vi "catch_block_on_floor.vi"() -> ()   [LabVIEW 2013]
panel:
  out "Voltage":dbl(graph)
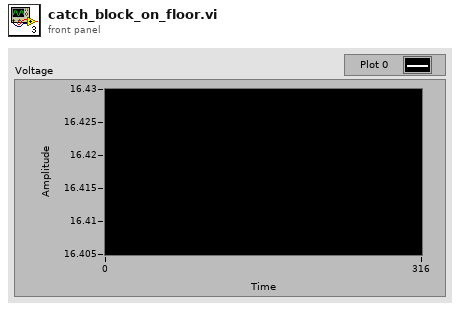
[diagram p1: front panel]
types:
  T1 = typedef "KNR3 Reference.ctl" = cluster{"FPGA Session":refnum<class "FPGA Interface Base.lvclass">, "Resource":T2}
  T2 = typedef "Resource.ctl" = enum16{"KNRm_DDRC", "KNRm_DDDD", "KNRm_DDDR", "KNRm_DDDC", "KNR"}
  T3 = cluster{"Mode":enum16{"FRWD", "TURFIX", "TURNOF"}, "Dir":enum16{"Left", "Right"}, "Pcmd":dbl, "Vcmd":dbl}
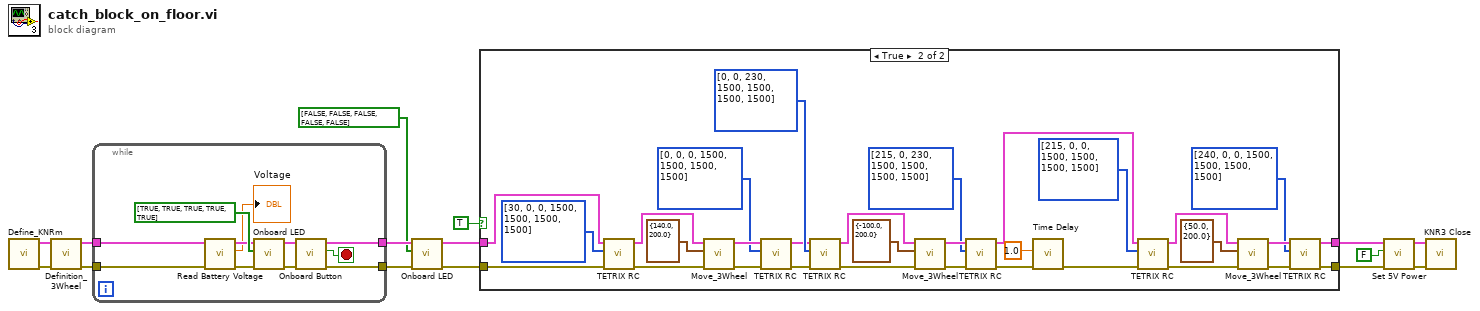
[diagram p0: block diagram]
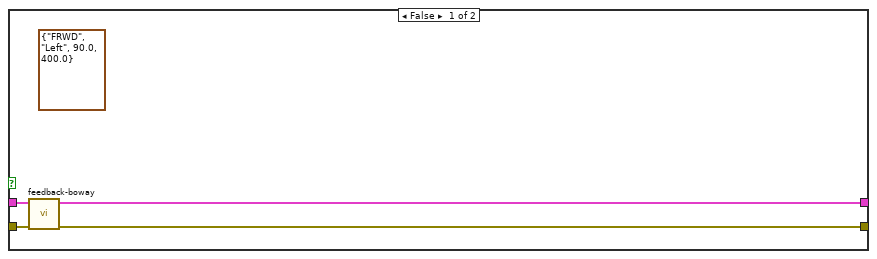
[diagram p2: hidden frame]
diagram:
  n1 = call "Define_KNRm.vi"() -> ("error out"=w6:errorcluster, "KNR out"=w7:T1)  [unwired: 10 in]
  n2 = call "Definition_3Wheel.vi"("error in (no error)"=w6, "KNR in"=w7) -> ("error out"=w8:errorcluster, "KNR out"=w9:T1)  [unwired: 8 in]
  n3 = while {
    tunnel: [w25] -> w15
    tunnel: [w23] -> w13
    tunnel: w9 -> [w18]
    tunnel: w8 -> [w17]
    stop <- w26 stop-if-true
    n4 = call <userlib>:"Read Battery Voltage.vi"("error in (no error)"=w17, "KNR in"=w18) -> ("error out"=w19:errorcluster, "Voltage"=→"Voltage":dbl, "KNR out"=w20:T1)  [unwired: 7 in]
    n5 = call <userlib>:"Onboard LED.vi"("error in (no error)"=w19, "LED List"=bool[] [TRUE, TRUE, TRUE, TRUE, TRUE], "KNR in"=w20) -> ("error out"=w24:errorcluster, "KNR out"=w22:T1)  [unwired: 7 in]
    n6 = call <userlib>:"Onboard Button.vi"("error in (no error)"=w24, "KNR in"=w22) -> ("error out"=w23:errorcluster, "value"=w26:bool, "KNR out"=w25:T1)  [unwired: 7 in]
  }
  n7 = call <userlib>:"Onboard LED.vi"("error in (no error)"=w13, "LED List"=bool[] [FALSE, FALSE, FALSE, FALSE, FALSE], "KNR in"=w15) -> ("error out"=w10:errorcluster, "KNR out"=w11:T1)  [unwired: 7 in]
  n8 = case shown="True" TRUE {
    tunnel: w10 -> [w30 w59]
    tunnel: [w29 w31] -> w1
    tunnel: w11 -> [w28 w60]
    tunnel: [w27 w32] -> w2
    frame False {
      (unwired) T3 {"Mode"=enum."FRWD", "Dir"=enum."Left", "Pcmd"=90.0, "Vcmd"=400.0} ("Move")
      n9 = call "feedback-boway.vi"("error in (no error)"=w30, "KNR in"=w28) -> ("error out"=w29:errorcluster, "KNR out"=w27:T1)  [unwired: 7 in, 1 out]
    }
    frame True {
      n10 = call "TETRIX RC.vi"("error in 2"=w59, "RC"=u16[] [30, 0, 0, 1500, 1500, 1500, 1500], "KNR in 3"=w60) -> ("error out 4"=w56:errorcluster, "KNR out 4"=w57:T1)  [unwired: 7 in]
      n11 = call "Move_3Wheel.vi"("error in (no error)"=w56, "Cluster"=cluster{"UDmm)":dbl, "Vcmd":dbl} {"UDmm)"=140.0, "Vcmd"=200.0}, "KNR in"=w57) -> ("error out"=w54:errorcluster, "KNR out"=w55:T1)  [unwired: 7 in]
      n12 = call "TETRIX RC.vi"("error in 2"=w54, "RC"=u16[] [0, 0, 0, 1500, 1500, 1500, 1500], "KNR in 3"=w55) -> ("error out 4"=w50:errorcluster, "KNR out 4"=w51:T1)  [unwired: 7 in]
      n13 = call "TETRIX RC.vi"("error in 2"=w50, "RC"=u16[] [0, 0, 230, 1500, 1500, 1500, 1500], "KNR in 3"=w51) -> ("error out 4"=w48:errorcluster, "KNR out 4"=w49:T1)  [unwired: 7 in]
      n14 = call "Move_3Wheel.vi"("error in (no error)"=w48, "Cluster"=cluster{"UDmm)":dbl, "Vcmd":dbl} {"UDmm)"=-100.0, "Vcmd"=200.0}, "KNR in"=w49) -> ("error out"=w46:errorcluster, "KNR out"=w45:T1)  [unwired: 7 in]
      n15 = call "TETRIX RC.vi"("error in 2"=w46, "RC"=u16[] [215, 0, 230, 1500, 1500, 1500, 1500], "KNR in 3"=w45) -> ("error out 4"=w41:errorcluster, "KNR out 4"=w39:T1)  [unwired: 7 in]
      n16 = call "Time Delay"("error in (no error)"=w41, "Delay Time (s)"=1.0) -> ("error out"=w40:errorcluster)  [unwired: 9 in]
      n17 = call "TETRIX RC.vi"("error in 2"=w40, "RC"=u16[] [215, 0, 0, 1500, 1500, 1500, 1500], "KNR in 3"=w39) -> ("error out 4"=w37:errorcluster, "KNR out 4"=w38:T1)  [unwired: 7 in]
      n18 = call "Move_3Wheel.vi"("error in (no error)"=w37, "Cluster"=cluster{"UDmm)":dbl, "Vcmd":dbl} {"UDmm)"=50.0, "Vcmd"=200.0}, "KNR in"=w38) -> ("error out"=w34:errorcluster, "KNR out"=w35:T1)  [unwired: 7 in]
      n19 = call "TETRIX RC.vi"("error in 2"=w34, "RC"=u16[] [240, 0, 0, 1500, 1500, 1500, 1500], "KNR in 3"=w35) -> ("error out 4"=w31:errorcluster, "KNR out 4"=w32:T1)  [unwired: 7 in]
    }
  }
  n20 = call <userlib>:"Set 5V Power.vi"("error in (no error)"=w1, "5V Power(T)"=FALSE, "KNR in"=w2) -> ("error out"=w4:errorcluster, "KNR out"=w5:T1)  [unwired: 7 in]
  n21 = call <userlib>:"KNR3 Close.vi"("error in (no error)"=w4, "KNR in"=w5) -> ()  [unwired: 9 in, 1 out]
